vi "Initialize Distance x Angle Vector.vi"(8 "Boolean":bool, 9 "First Index":i32, 10 "Num_Points_Scan":u16, 11 "Distance x Angle In":cluster{"Magnitude":dbl, "Phase":dbl}[](array[cluster])) -> (3 "Distance x Angule":cluster{"Magnitude":dbl, "Phase":dbl}[](array[cluster]))   [LabVIEW 2019, in "PF_API.lvclass"]
uses:
  PF_API.lvclass
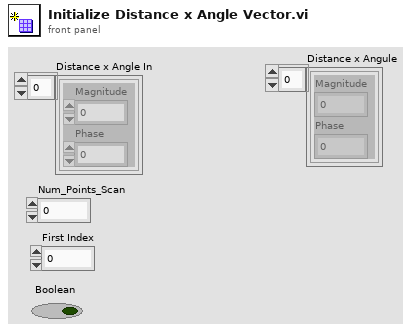
[diagram p1: front panel]
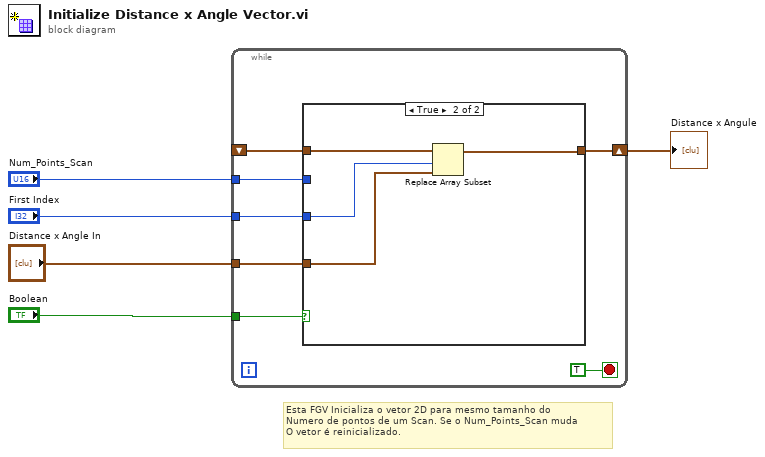
[diagram p0: block diagram]
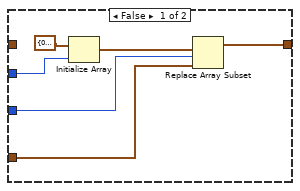
[diagram p2: hidden frame]
diagram:
  # "Esta FGV Inicializa o vetor 2D para mesmo tamanho do\nNumero de pontos de um Scan. Se o Num_Points_Scan muda\nO vetor é reinicializado."
  n1 = while {
    tunnel: "Num_Points_Scan" -> [w11]
    tunnel: "Boolean" -> [w10]
    shift-right: [w12] -> w3
    shift-left: _ -> [w9]
    tunnel: "Distance x Angle In" -> [w7]
    tunnel: "First Index" -> [w6]
    stop <- TRUE stop-if-true
    n2 = case shown="True" w10 {
      tunnel: w11 -> [w17 _]
      tunnel: [w14 w20] -> w12
      tunnel: w9 -> [_ w22]
      tunnel: w7 -> [w15 w21]
      tunnel: w6 -> [w13 w19]
      frame False {
        n3 = Initialize Array(cluster{"Magnitude":dbl, "Phase":dbl} {"Magnitude"=0.0, "Phase"=0.0}, w17) -> (w16:cluster{"Magnitude":dbl, "Phase":dbl}[])
        n4 = Replace Array Subset(array=w16, new element=w15, index=w13) -> (w14:cluster{"Magnitude":dbl, "Phase":dbl}[])
      }
      frame True {
        n5 = Replace Array Subset(array=w22, new element=w21, index=w19) -> (w20:cluster{"Magnitude":dbl, "Phase":dbl}[])
      }
    }
  }
  "Distance x Angule" <- w3
